vi "ReadInHeightSurvey.vi"(1 "VP.TTHeightCorrs In":T1={"TT.Azimuths"=[10.0, 30.0, 50.0, 70.0, 90.0, 110.0, 130.0, 150.0, 170.0, 190.0, 210.0, 230.0, 250.0, 270.0, 290.0, 310.0, 330.0, 350.0], "Z.HeightCorrs"=[[0.1, 0.05], [0.05, 0.05], [0.0, 1.0], [-0.1, 2.65], [-1.0, 3.8000000000000003], [-1.9, 5.35], [-2.5, 7.05], [-3.45, 8.3], [-4.2, 9.4], [-4.7, 9.75], [-5.05, 9.2], [-4.8, 8.5], [-4.15, 7.35], [-3.55, 5.4], [-2.75, 3.55], [-1.65, 2.15], [-0.8, 0.7], [-0.25, -0.05], [2.4, 0.0], [2.5, 0.0], [2.5, 0.0], [2.2, 0.0], [1.3, 0.0], [0.7, 0.0], [0.4, 0.0], [0.0, 0.0], [0.0, 0.0], [0.8, 0.0], [1.1, 0.0], [1.7, 0.0], [2.4, 0.0], [2.4, 0.0], [2.3, 0.0], [2.3, 0.0], [1.2, 0.0], [0.4, 0.0]], "Use Height Corrections"=TRUE, "Height Survey Filepaths"=[], "Corrections from File"=TRUE}) -> (0 "VP.TTHeightCorrs Out":T1={"TT.Azimuths"=[10.0, 30.0, 50.0, 70.0, 90.0, 110.0, 130.0, 150.0, 170.0, 190.0, 210.0, 230.0, 250.0, 270.0, 290.0, 310.0, 330.0, 350.0], "Z.HeightCorrs"=[[0.1, 0.05], [0.05, 0.05], [0.0, 1.0], [-0.1, 2.65], [-1.0, 3.8000000000000003], [-1.9, 5.35], [-2.5, 7.05], [-3.45, 8.3], [-4.2, 9.4], [-4.7, 9.75], [-5.05, 9.2], [-4.8, 8.5], [-4.15, 7.35], [-3.55, 5.4], [-2.75, 3.55], [-1.65, 2.15], [-0.8, 0.7], [-0.25, -0.05], [2.4, 0.0], [2.5, 0.0], [2.5, 0.0], [2.2, 0.0], [1.3, 0.0], [0.7, 0.0], [0.4, 0.0], [0.0, 0.0], [0.0, 0.0], [0.8, 0.0], [1.1, 0.0], [1.7, 0.0], [2.4, 0.0], [2.4, 0.0], [2.3, 0.0], [2.3, 0.0], [1.2, 0.0], [0.4, 0.0]], "Use Height Corrections"=TRUE, "Height Survey Filepaths"=[], "Corrections from File"=TRUE})   [LabVIEW 2015]
uses:
  <vilib>/Utility/file.llb/Read Delimited Spreadsheet (DBL).vi
panel:
  out "Height Survey File Data":dbl[][](array[numeric])
  # "<Column 1> TurnTable Azimuth [deg]\n<Column 2> X [mm]\n<Column 3> Y [mm]\n<Column 4> Z [mm]\n<Column 5> Zsensor [mm]"
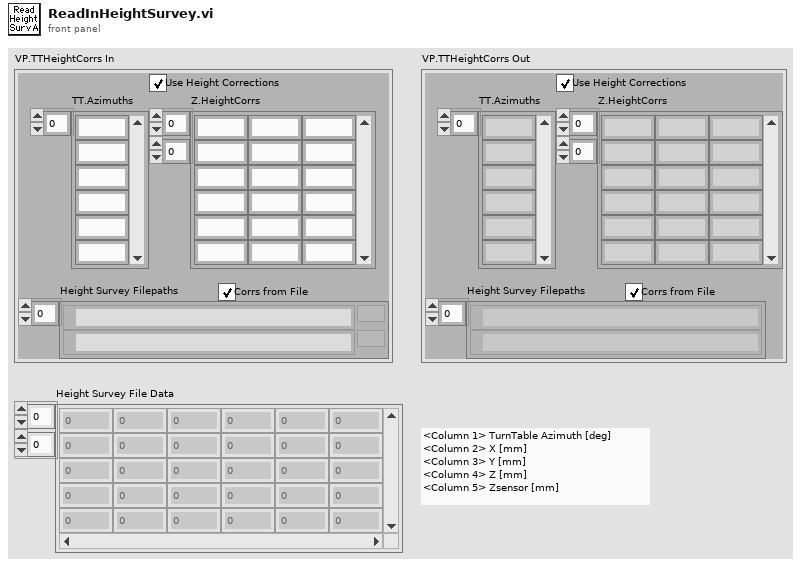
[diagram p1: front panel]
types:
  T1 = cluster{"TT.Azimuths":dbl[], "Z.HeightCorrs":dbl[][], "Use Height Corrections":bool, "Height Survey Filepaths":path[], "Corrections from File":bool}
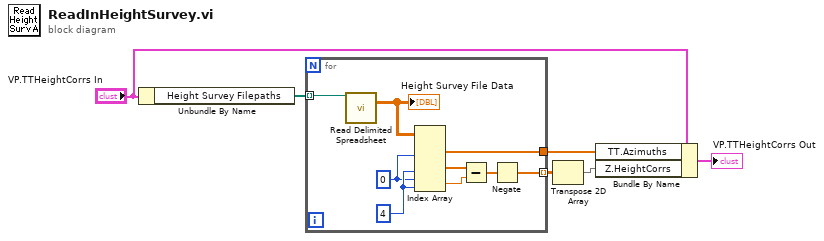
[diagram p0: block diagram]
diagram:
  n1 = Unbundle By Name("VP.TTHeightCorrs In") -> ("Height Survey Filepaths"=w3:path[])
  n2 = for {
    tunnel: w3 -> [w15] mode=indexing
    tunnel: [w13] -> w6
    tunnel: [w8] -> w4 mode=indexing
    w12 = 4 ("index (col)")
    w7 = 0 ("disabled index (col)")
    n3 = call-poly <vilib>:"Read Delimited Spreadsheet.vi"("file path (dialog if empty)"=w15) -> ("all rows"=w14:dbl[][])  [unwired: 9 in, 5 out]
    "Height Survey File Data" <- w14
    n4 = Index Array(array=w14, index (col) #1=w7, index (col) #2=w12, index (row) #3=w7, index (col) #3=w12) -> (element #1=w13:dbl[], element #2=w11:dbl[], element #3=w10:dbl)  [unwired: 2 in]
    n5 = Subtract(x=w11, y=w10) -> (x-y=w9:dbl[])
    n6 = Negate(x=w9) -> (-x=w8:dbl[])
  }
  n7 = Transpose 2D Array(2D array=w4) -> (transposed array=w5:dbl[][])
  n8 = Bundle By Name(cluster="VP.TTHeightCorrs In", "TT.Azimuths"=w6, "Z.HeightCorrs"=w5) -> (→"VP.TTHeightCorrs Out":T1)
